vi "Vision.vi"() -> ()   [LabVIEW 2013]
uses:
  StateMachineStates 1.ctl
  <vilib>/DAQmx/read.llb/DAQmx Read (Counter DBL 1Chan 1Samp).vi
  <vilib>/Utility/file.llb/Write To Spreadsheet File (DBL).vi
  <vilib>/DAQmx/create/channels.llb/DAQmx Create Channel (CI-Pulse Width).vi
  <vilib>/DAQmx/miscellaneous.llb/DAQmx Fill In Error Info.vi
panel:
  in  "Stimulus delay (ms)":u32
  in  "N \n(calibration)":i32=5
  in  "Threshold\n (calibration)":dbl
  out "Pump calibration array":dbl[][](array[numeric])
  out "Calibrating":bool
  in  "Calibrate":bool
  out "current time":timestamp
  in  "Threshold":dbl=0.1 format="%#_13g"
  in  "Number of\ntrials to avg":i32=5
  in  "Pump mode":enum16{"Constant power", "Constant time"}(ring)
  in  "Target trigger\nrate (Hz)":dbl
  out "Pockels cell\nposition":dbl
  out "Waveplate\nposition":dbl
  out "Right\nposition":dbl
  out "Left\nposition":dbl
  in  "EEG timeout":i32
  out "Triggered":bool
  in  "Use EEG trigger?":bool
  in  "Entrainment":bool
  in  "Sound at \nstimulus end":bool
  in  "Manual \nvoltage (V)":dbl=2.6 format="%.2p"
  in  "Manual \nphoton #":i64=100
  out "L/R WP target":dbl
  out "List of axes":i32[](array[numeric])
  out "List of WP errors":bool[](array[boolean])
  out "WP error":bool
  out "appended array":dbl[][](array[numeric])
  out "Pump WP":dbl format="%.2f"
  in  "Target trial \nlength (ms)":dbl=500.0 format="%.2p"
  in  "Default pump \nWP angle":dbl=52.6
  in  "Pump WP":bool
  out "Photon time (ms)":dbl format="%.2f"
  in  "Interval (ms)":u32
  out "Repetition":dbl
  in  "Repetitions":dbl=1.0
  out "WP time (ms)":u32
  out "VISA Handle out":refnum<visa-resource-name>="ASRL5::INSTR"
  out "Initializing":bool
  out "Trial mode":enum16{"Single Photons", "LED", "Mixed LED"}(ring)
  in  "Frequency of LED trials\nfor Mixed mode":dbl=30.0
  out "Bright trial\nrequested":bool
  out "Observer Ready":bool
  in  "Bright/mixed mode \nLED voltage (V)":dbl=2.6 min=-3.0 max=4.0 format="%.2f"
  in  "GPIB address":string="15"
  in  "Period (ms)":i64=20
  in  "Pulse \nlength (ms)":dbl=50.0
  out "L/R WP":dbl format="%.2f"
  in  "Manually \ninitialize":bool
  in  "COM for WPs":u8=3
  out "Blocked trial #":i32
  out "Photon #":i32
  out "LED Voltage":dbl
  in  "Blocking requirements":cluster{"Value":dbl, " Number":i32}[](array[cluster])
  in  "Manual":bool
  in  "Path":path=path "C:/Users/lab/Dropbox/Research/Data/Vision"
  out "Counts 2":u32
  out "Counts 1":u32
  in  "Delay for APDs (ms)":u32
  in  "Counter 2":tag="Dev1/ctr1"
  in  "Counter 1":tag="Dev1/ctr0"
  out "Trial #":i32
  in  "Session Mode":enum16{"Single Photons", "LED", "Mixed"}(ring)=enum."Mixed"
  in  "Audio":bool=TRUE
  in  "Self-paced":bool
  out "Stimulus":bool
  out "Location Set":bool
  out "Stimulus \nlocation":string
  out "Waiting":bool
  out "Observer Responded":bool
  out "Response \ntime (ms)":dbl
  out "Observer \nchoice":string
  out "Confidence":i32
  in  "stop":bool
  in  "Next Trial":bool
  in  "Create New File":bool
  out "Subject #":string
  # "Instructions: Run VI. Enter blocking requirements, then press\nCreate New File. Initialize waveplates if necessary, and set\nhighlighted controls to desired values. Press Next Trial to begin."
  # "Researcher Interface"
  # "Settings for Blocking\nand Mixed Mode"
  # "(1)"
  # "Trial Options"
  # "Counter Options"
  # "Trial Information"
  # "EEG Options"
  # "Pump Settings"
  # "Waveplates"
  # "LED Options"
  # "(3)"
  # "(2)"
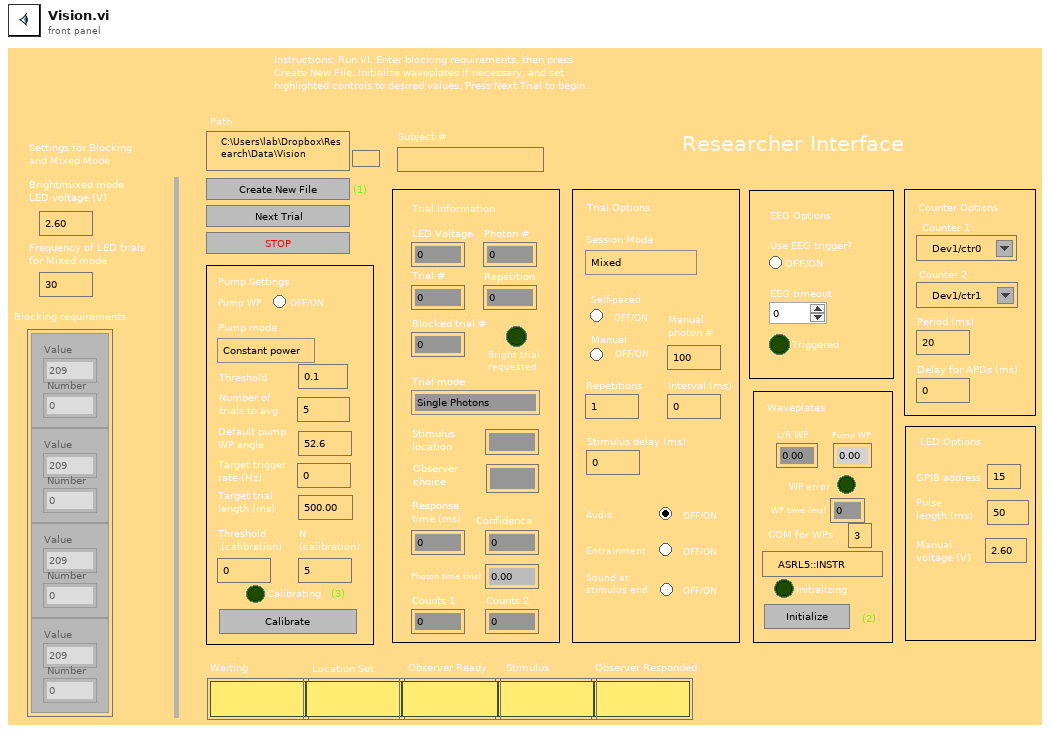
[diagram p1: front panel]
types:
  T1 = typedef "StateMachineStates 1.ctl" = enum16{"WaitResearcher", "Setup", "SetWP", "WaveplateError", "WaitObserverReady", "EEG", "Photons", "LED", "WaitObserverResponse", "CleanUp", "Stop"}
  T2 = enum16{"0", "1", "2", "3", "4", "5", "6", "7", "8", "9", "A", "B", "C", "D", "E", "F", "G", "H", "I", "J", "K", "L", "M", "N", "O", "P", "Q", "R", "S", "T", "U", "V", "W", "X", "Y", "Z", "F1", "F2", "F3", "F4", "F5", "F6", "F7", "F8", "F9", "F10", "F11", "F12", "F13", "F14", "F15", "ADD", "BACK", "BACKSLASH", "CAPITAL", "COMMA", "DECIMAL", "DELETE", "DIVIDE", "DOWN", "END", "EQUALS", "ESCAPE", "GRAVE (`)", "HOME", "INSERT", "LBRACKET", "LCONTROL", "LEFT", "L ALT", "LSHIFT", "LWIN", "MINUS", "MULTIPLY", "NEXT", "NUMLOCK", "NUMPAD_0", "NUMPAD_1", "NUMPAD_2", "NUMPAD_3", "NUMPAD_4", "NUMPAD_5", "NUMPAD_6", "NUMPAD_7", "NUMPAD_8", "NUMPAD_9", "PAUSE", "PERIOD", "PRIOR (PG UP)", "RBRACKET", "RCONTROL", "RETURN", "RIGHT", "R ALT", "RSHIFT", "RWIN", "SCROLL", "SEMICOLON", "SLASH", "SPACE", "SUBTRACT", "TAB", "UP", "ENTER (num pad)", "' (quote)"}
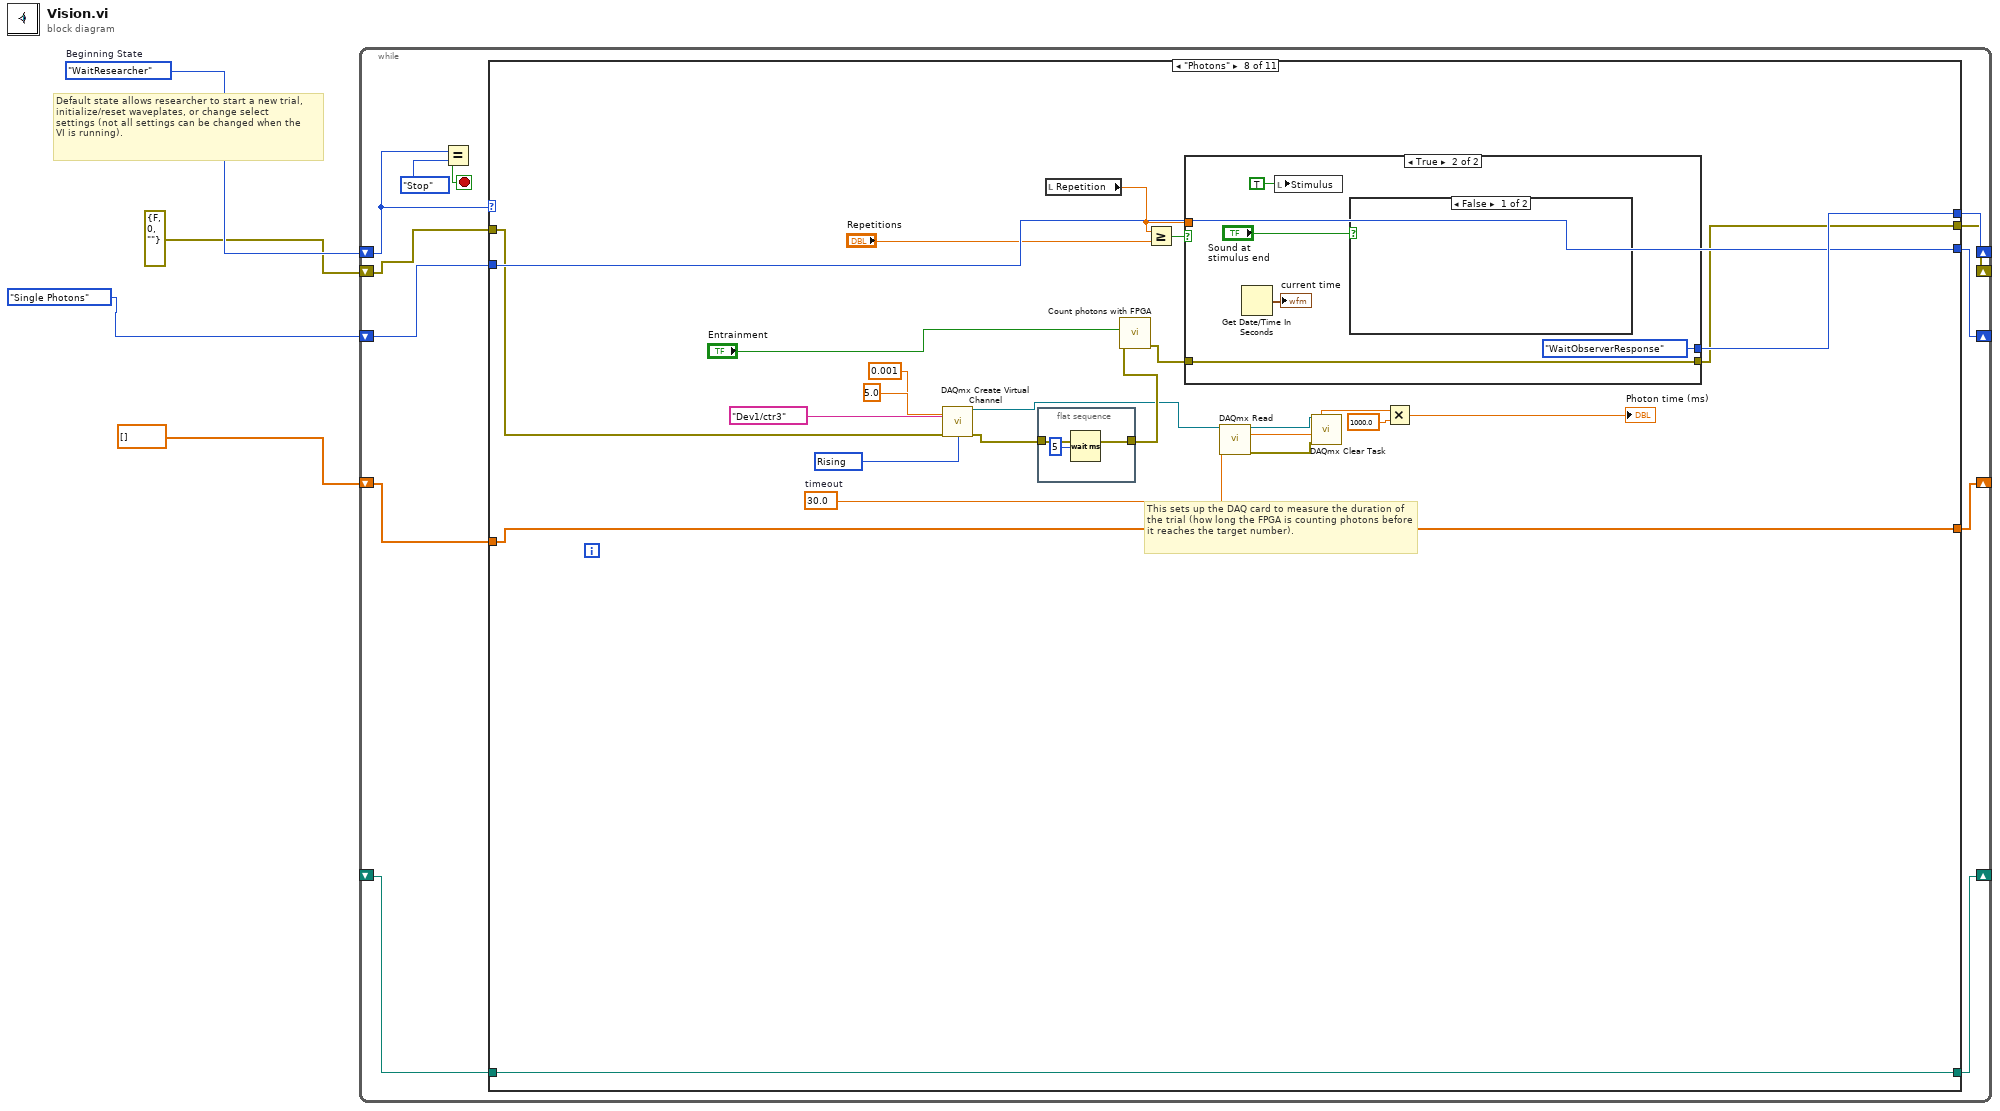
[diagram p0: block diagram]
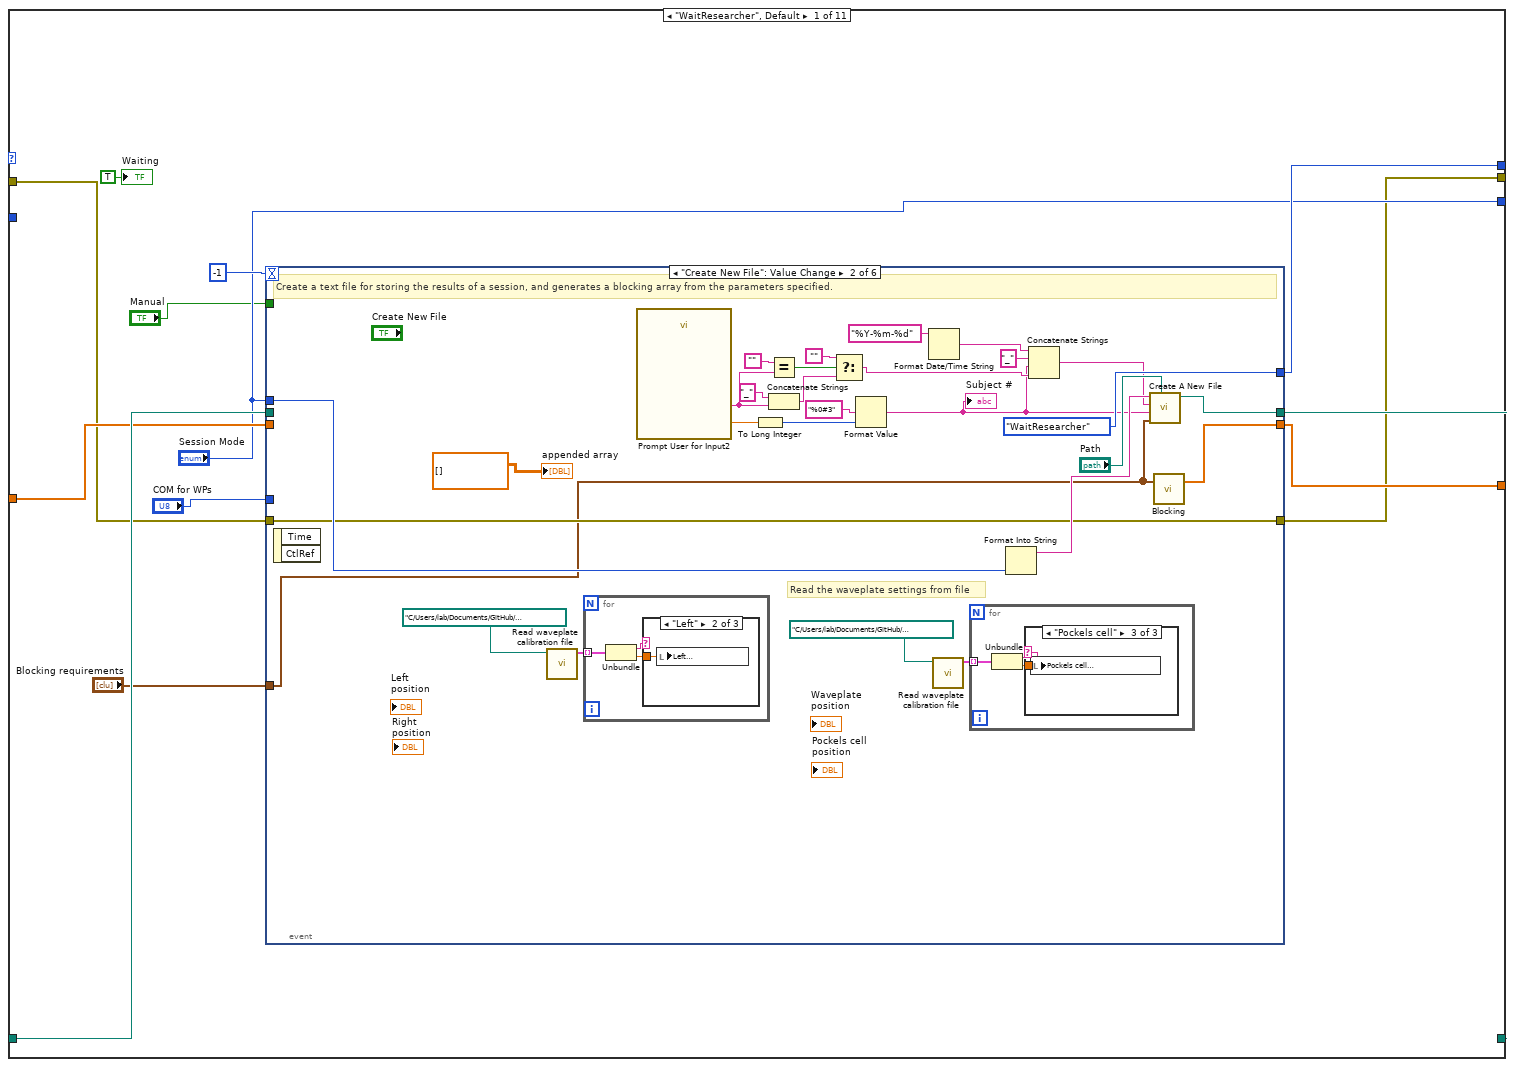
[diagram p2: hidden frame]
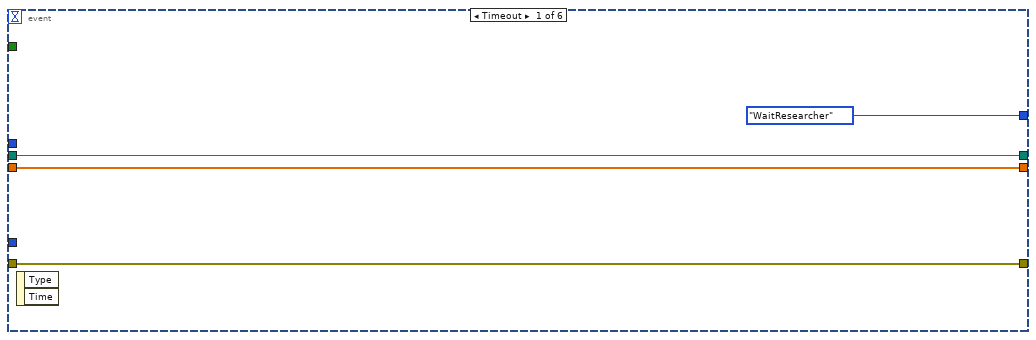
[diagram p3: hidden frame]
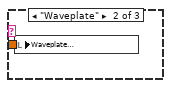
[diagram p5: hidden frame]
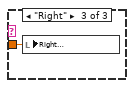
[diagram p7: hidden frame]
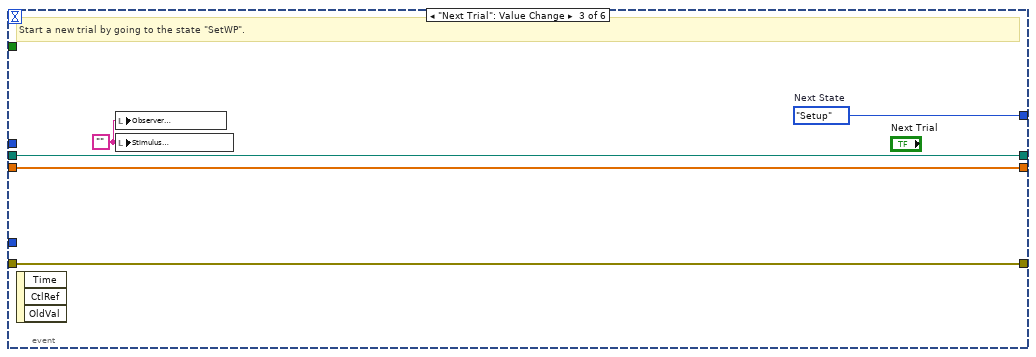
[diagram p8: hidden frame]
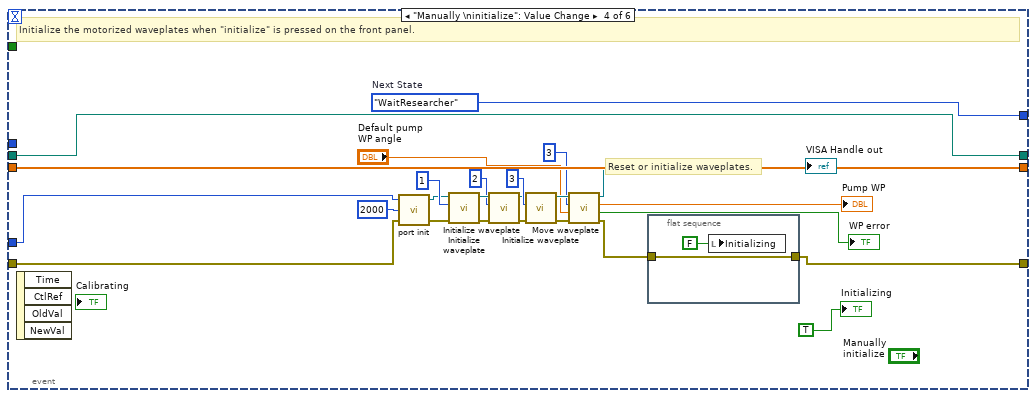
[diagram p9: hidden frame]
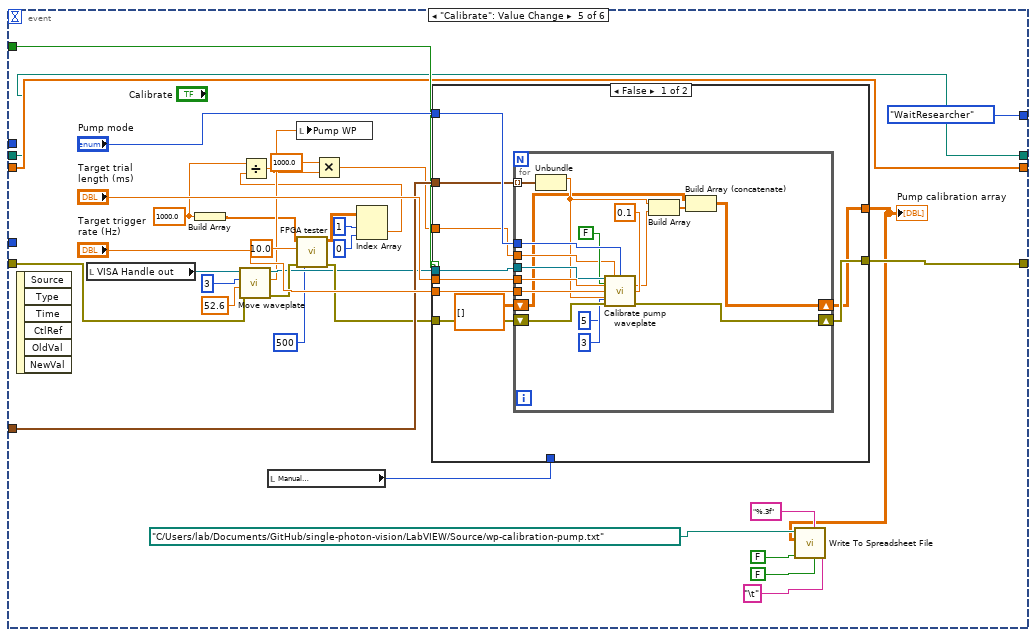
[diagram p10: hidden frame]
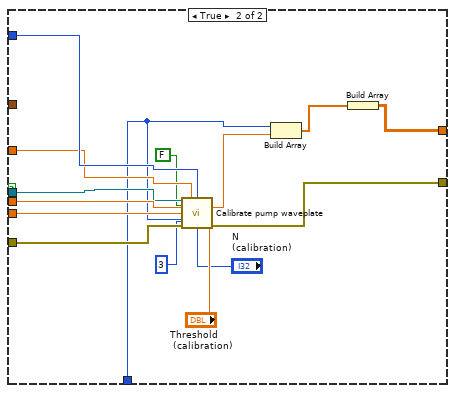
[diagram p11: hidden frame]
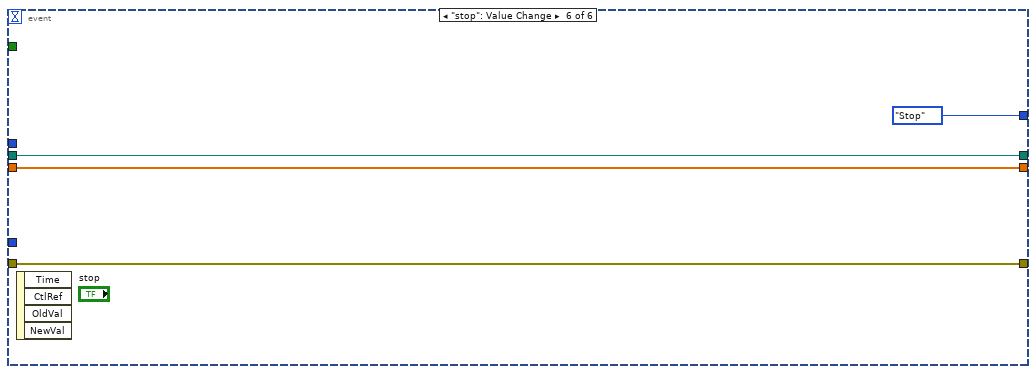
[diagram p12: hidden frame]
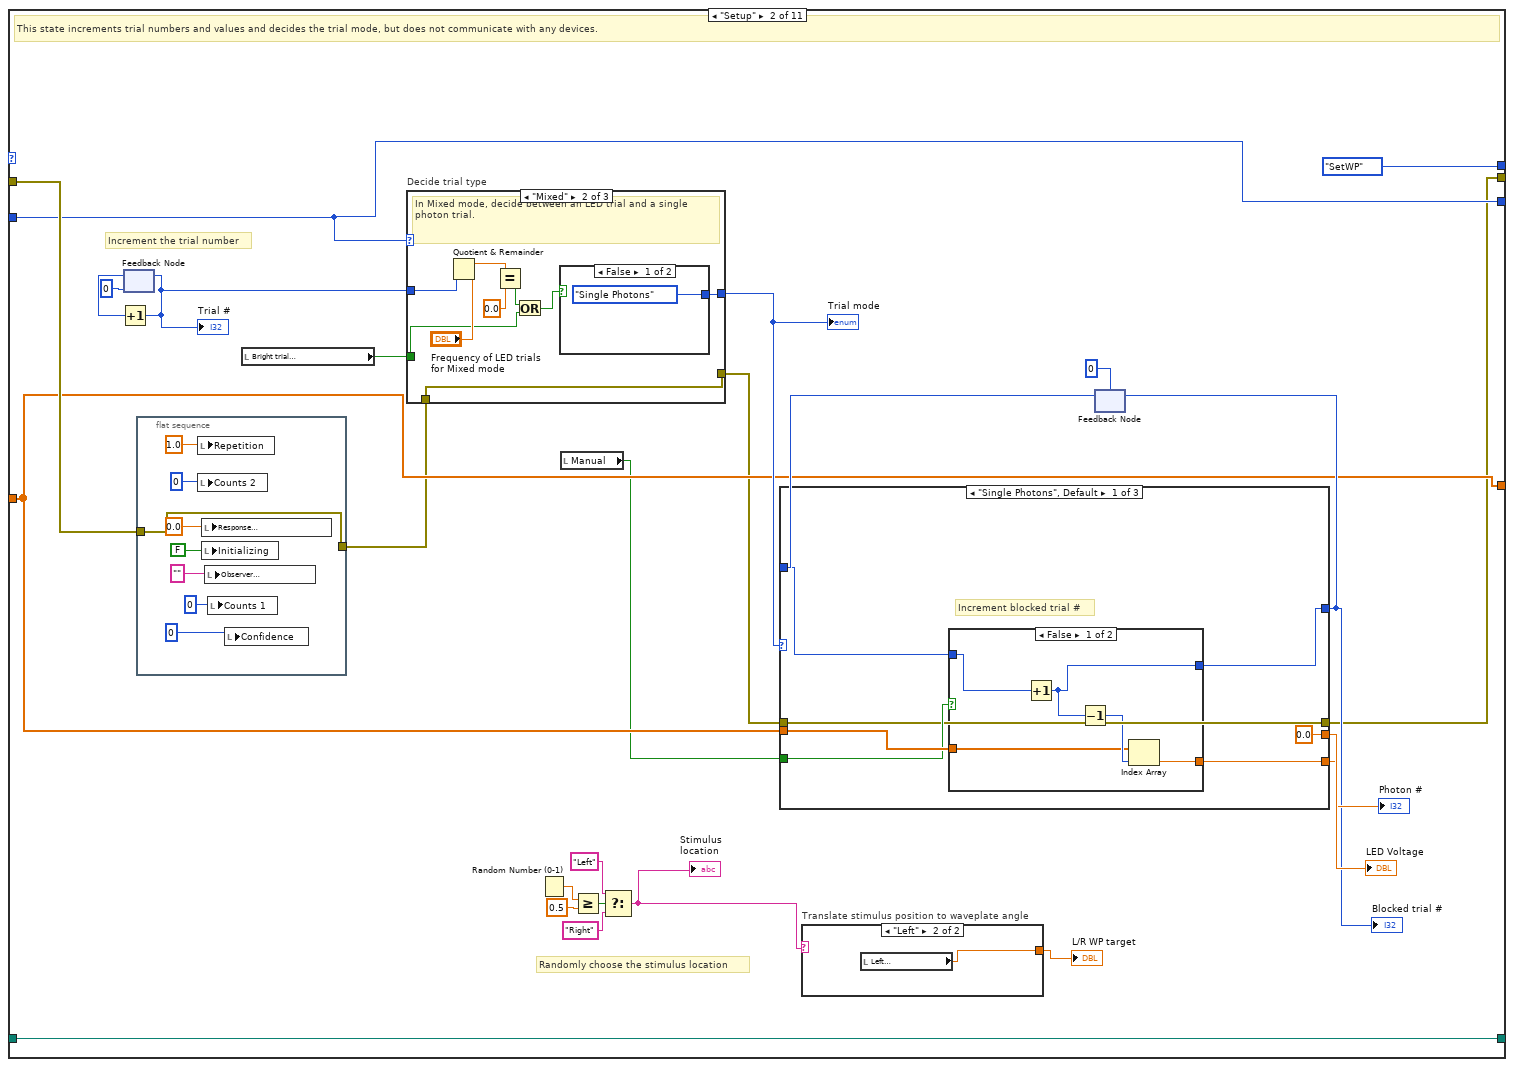
[diagram p13: hidden frame]
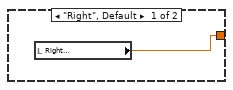
[diagram p14: hidden frame]
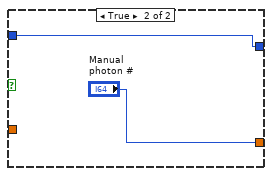
[diagram p15: hidden frame]
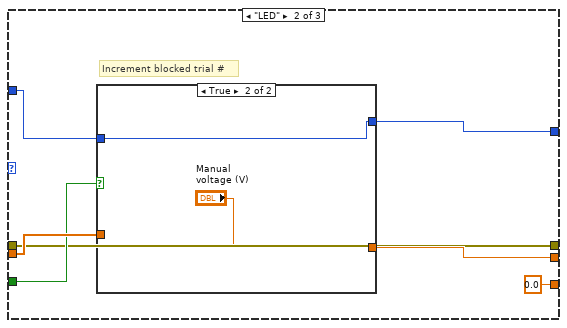
[diagram p16: hidden frame]
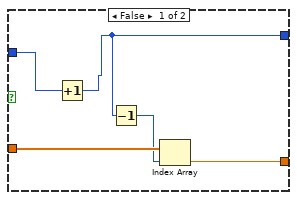
[diagram p17: hidden frame]
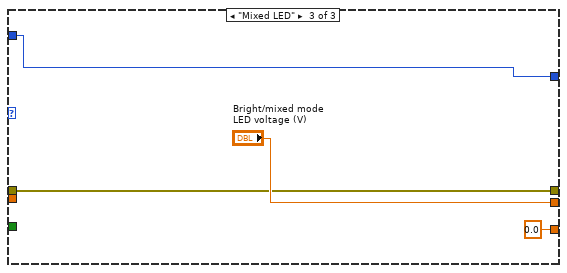
[diagram p18: hidden frame]
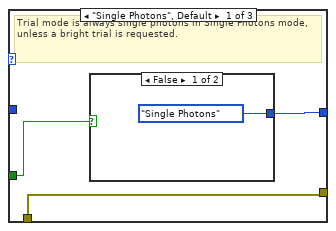
[diagram p19: hidden frame]
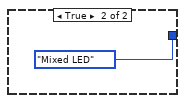
[diagram p20: hidden frame]
diagram:
  w4 = StateMachineStates_1."WaitResearcher"  # Beginning State
  # "Default state allows researcher to start a new trial,\ninitialize/reset waveplates, or change select\nsettings (not all settings can be changed when the\nVI is running)."
  n1 = while {
    shift-right: [w13] -> _
    shift-left: w4 -> [w14]
    shift-right: [w6] -> _
    shift-left: errorcluster {"status"=FALSE, "code"=0, "source"=""} ("error out") -> [w12]
    shift-right: [w11] -> _
    shift-left: enum16{"Single Photons", "LED", "Mixed"}."Single Photons" ("Mode") -> [w10]
    shift-right: [w9] -> _
    shift-left: _ -> [w5]
    shift-right: [w8] -> _
    shift-left: dbl[] [] ("Blocking array") -> [w7]
    stop <- w16 stop-if-true
    n2 = Equal?(x=w14, y=StateMachineStates_1."Stop" ("States")) -> (x = y?=w16:bool)
    n3 = case shown="\"Photons\"" w14 {
      selector: w14 -> [_ _ _ _ w497 _ _ _ _ _ _]
      tunnel: [w29 StateMachineStates_1."SetWP" ("Next State") w301 w443 w498 w539 StateMachineStates_1."WaitObserverResponse" ("Next State") w593 w610 w666 w705] -> w13
      tunnel: [w20 w193 w281 w440 w490 w541 w566 w589 w611 w657 w709] -> w6
      tunnel: w12 -> [w21 w210 w307 w444 w491 w541 w555 w575 w612 w656 w708]
      tunnel: ["Session Mode" w199 w319 w447 w495 w542 w562 w592 w617 w664 w712] -> w11
      tunnel: w10 -> [_ w199 w319 w447 w494 w542 w562 w592 w617 w664 w712]
      tunnel: [w26 w192 w320 w445 w493 w543 w559 w591 w616 w663 w711] -> w9
      tunnel: w5 -> [w25 w192 w320 w445 w493 w543 w559 w591 w616 w663 w711]
      tunnel: [w24 w198 w310 w446 w492 w544 w558 w590 w615 w661 w710] -> w8
      tunnel: w7 -> [w23 w198 w310 w446 w492 w544 w558 w590 w615 w661 w710]
      frame "WaitResearcher", Default {
        n4 = event shown="[1] \"Create New File\": Value Change" {
          selector: _ -> [_ _ _ _ _ _]
          dyn-events: _ -> [_ _ _ _ _ _]
          timeout: -1 -> [_ _ _ _ _ _]
          tunnel: [StateMachineStates_1."WaitResearcher" ("Next State") StateMachineStates_1."WaitResearcher" ("Next State") w72 w101 StateMachineStates_1."WaitResearcher" ("Next State") StateMachineStates_1."Stop" ("Next State")] -> w29
          tunnel: "Session Mode" -> [_ w57 _ _ _ _]
          tunnel: [w33 w52 w75 w100 w106 w183] -> w26
          tunnel: w25 -> [w33 _ w75 w100 w106 w183]
          tunnel: [w32 w55 w74 w98 w107 w182] -> w24
          tunnel: w23 -> [w32 _ w74 w98 w107 w182]
          tunnel: w21 -> [w31 w51 w73 w93 w128 w181]
          tunnel: [w31 w51 w73 w97 w134 w181] -> w20
          tunnel: "COM for WPs" -> [_ _ _ w94 _ _]
          tunnel: "Blocking requirements" -> [_ w34 _ _ w135 _]
          tunnel: "Manual" -> [_ _ _ _ w121 _]
          event Timeout {
            n5 = event-data() -> ()  [unwired: 1 in, 2 out]
          }
          event "Create New File": Value Change {
            # "Read the waveplate settings from file"
            # "Create a text file for storing the results of a session, and generates a blocking array from the parameters specified."
            n6 = event-data() -> ()  [unwired: 1 in, 2 out]
            n7 = call "Read waveplate calibration file.vi"("file path (dialog if empty)"=path "C:/Users/lab/Documents/GitHub/single-photon-vision/LabVIEW/Source/wp-calibration-lr.txt") -> ("Calibration array"=w37:cluster{"String":string, dbl}[])  [unwired: 9 in, 1 out]
            n8 = for {
              tunnel: w37 -> [w69] mode=indexing
              n9 = Unbundle(w69) -> ("String"=w68:string, w67:dbl)
              n10 = case shown="\"Left\"" w68 {
                tunnel: w67 -> [_ w70 w71]
                frame Default {
                }
                frame "Left" {
                  n11 = local write "Left\nposition"(w70) -> ()
                }
                frame "Right" {
                  n12 = local write "Right\nposition"(w71) -> ()
                }
              }
            }
            n13 = call "Prompt User for Input2"() -> ("Subject #"=w60:dbl, "Filename"=w46:string)  [unwired: 16 in, 2 out]
            n14 = To Long Integer(number=w60) -> (32bit integer=w42:i32)
            n15 = Equal?(x="", y=w46) -> (x = y?=w58:bool)
            n16 = Concatenate Strings("_" ("string"), w46) -> (w49:string)
            n17 = Select(t="", s=w58, f=w49) -> (s? t:f=w44:string)
            n18 = Format Value(format string="%0#3", value (0)=w42) -> (output string=w41:string)  [unwired: 1 in]
            "Subject #" <- w41
            n19 = Format Date/Time String(time format string (%c)="%Y-%m-%d") -> (date/time string=w47:string)  [unwired: 2 in]
            n20 = call "Read waveplate calibration file.vi"("file path (dialog if empty)"=path "C:/Users/lab/Documents/GitHub/single-photon-vision/LabVIEW/Source/wp-calibration-pc.txt") -> ("Calibration array"=w35:cluster{"String":string, dbl}[])  [unwired: 9 in, 1 out]
            n21 = for {
              tunnel: w35 -> [w64] mode=indexing
              n22 = Unbundle(w64) -> ("String"=w63:string, w62:dbl)
              n23 = case shown="\"Pockels cell\"" w63 {
                tunnel: w62 -> [_ w65 w66]
                frame Default {
                }
                frame "Waveplate" {
                  n24 = local write "Waveplate\nposition"(w65) -> ()
                }
                frame "Pockels cell" {
                  n25 = local write "Pockels cell\nposition"(w66) -> ()
                }
              }
            }
            n26 = Format Into String(w57) -> (resulting string=w56:string)  [unwired: 3 in, 1 out]
            n27 = Concatenate Strings(w47, "_" ("string"), w41, w44) -> (w53:string)
            n28 = call "Create A New File.vi"("Path in"="Path", "Blocking requirements"=w34, "Subject #"=w41, "Filename"=w53, "Mode"=w56) -> ("Path out"=w52:path)  [unwired: 6 in]
            n29 = call "Blocking.vi"("Blocking requirements"=w34) -> ("Blocking array"=w55:dbl[])  [unwired: 2 in]
            "appended array" <- dbl[][] []
          }
          event "Next Trial": Value Change {
            w72 = StateMachineStates_1."Setup"  # Next State
            w76 = ""
            # "Start a new trial by going to the state \"SetWP\"."
            n30 = event-data() -> ()  [unwired: 1 in, 3 out]
            n31 = local write "Observer \nchoice"(w76) -> ()
            n32 = local write "Stimulus \nlocation"(w76) -> ()
          }
          event "Manually \ninitialize": Value Change {
            w101 = StateMachineStates_1."WaitResearcher"  # Next State
            # "Reset or initialize waveplates."
            # "Initialize the motorized waveplates when \"initialize\" is pressed on the front panel."
            n33 = event-data() -> ()  [unwired: 1 in, 4 out]
            n34 = call "port init.vi"("error in"=w93, "Timeout (ms)"=u32 2000 ("Timeout (300 ms)"), "SerialPort"=w94) -> ("error out"=w92:errorcluster, "Visa Handle"=w91:refnum<visa-resource-name>)  [unwired: 1 in]
            n35 = call "Initialize waveplate.vi"("error in (no error)"=w92, "Axis in"=1, "VISA Handle in"=w91) -> ("error out"=w88:errorcluster, "VISA Refnum out"=w90:refnum<visa-resource-name>)  [unwired: 6 in, 1 out]
            n36 = call "Initialize waveplate.vi"("error in (no error)"=w88, "Axis in"=2, "VISA Handle in"=w90) -> ("error out"=w85:errorcluster, "VISA Refnum out"=w86:refnum<visa-resource-name>)  [unwired: 6 in, 1 out]
            n37 = call "Initialize waveplate.vi"("error in (no error)"=w85, "Axis in"=3, "VISA Handle in"=w86) -> ("error out"=w81:errorcluster, "VISA Refnum out"=w84:refnum<visa-resource-name>)  [unwired: 6 in, 1 out]
            n38 = call "Move waveplate.vi"("error in (no error)"=w81, "Angle"="Default pump \nWP angle", "Axis in"=3, "VISA Refnum in"=w84) -> ("error out"=w80:errorcluster, "WP Error"=→"WP error":bool, "Current position (units)"=→"Pump WP":dbl, "VISA Refnum out"=→"VISA Handle out":refnum<visa-resource-name>)  [unwired: 4 in]
            n39 = flat-sequence {
              tunnel: w80 -> [w103]
              tunnel: [w103] -> w97
              frame #0 {
                n40 = local write "Initializing"(FALSE ("Initializing waveplates")) -> ()
              }
            }
            "Initializing" <- TRUE ("Initializing waveplates")
          }
          event "Calibrate": Value Change {
            w113 = 1000.0 ("element")
            n41 = event-data() -> ()  [unwired: 1 in, 6 out]
            n42 = local read "VISA Handle out"() -> (w126:refnum<visa-resource-name>)
            n43 = Build Array(w113) -> (w114:dbl[])
            n44 = call "Move waveplate.vi"("error in (no error)"=w128, "Angle"=52.6, "Axis in"=3, "VISA Refnum in"=w126) -> ("error out"=w127:errorcluster, "Current position (units)"=w122:dbl, "VISA Refnum out"=w125:refnum<visa-resource-name>)  [unwired: 4 in, 1 out]
            n45 = local read "Manual \nphoton #"() -> (w120:i64)
            n46 = local write "Pump WP"(w122) -> ()
            n47 = call "FPGA tester.vi"("error in"=w127, "Delay"=u32 500, "Repetitions"=10.0, "Levels"=w114) -> ("error out"=w133:errorcluster, "Results"=w131:dbl[][])  [unwired: 2 in]
            n48 = Index Array(array=w131, index (row)=1, index (col)=0 ("disabled index (col)")) -> (element=w112:dbl)
            n49 = Divide(x=w113, y=w112) -> (x/y=w111:dbl)
            n50 = Multiply(x=1000.0, y=w111) -> (x*y=w109:dbl)
            n51 = case shown="False" w121 {
              tunnel: "Target trigger\nrate (Hz)" -> [w148 w180]
              tunnel: "Target trial \nlength (ms)" -> [w147 w179]
              tunnel: "Pump mode" -> [w146 w178]
              tunnel: w135 -> [w145 _]
              tunnel: [w144 w177] -> w134
              tunnel: w133 -> [w143 w176]
              tunnel: w109 -> [w142 w175]
              tunnel: w125 -> [w141 w174]
              tunnel: w120 -> [_ w173]
              tunnel: [w140 w168] -> w108
              frame False {
                n52 = for {
                  tunnel: w148 -> [w165]
                  tunnel: w147 -> [w164]
                  tunnel: w146 -> [w163]
                  tunnel: w145 -> [w162] mode=indexing
                  shift-right: [w160] -> w144
                  shift-left: w143 -> [w161]
                  tunnel: w141 -> [w159]
                  tunnel: w142 -> [w154]
                  shift-right: [w150] -> w140
                  shift-left: dbl[][] [] -> [w149]
                  n53 = Unbundle(w162) -> ("Value"=w153:dbl)  [unwired: 1 out]
                  n54 = call "Calibrate pump waveplate.vi"("VISA Refnum in"=w159, "Trigger rate \nat maximum"=w154, "Mode"=w163, "Trigger rate warnings?"=FALSE, "Target trial \nlength (ms)"=w164, "Target trigger rate"=w165, "Threshold"=0.1, "Photon #"=w153, "error in (no error)"=w161, "N"=5, "Axis in"=3) -> ("WP position"=w152:dbl, "error out"=w160:errorcluster)  [unwired: 1 in, 2 out]
                  n55 = Build Array(w153, w152) -> (w151:dbl[])
                  n56 = Build Array (concatenate)(w149, w151) -> (w150:dbl[][])
                }
              }
              frame True {
                n57 = call "Calibrate pump waveplate.vi"("VISA Refnum in"=w174, "Trigger rate \nat maximum"=w175, "Mode"=w178, "Trigger rate warnings?"=FALSE, "Target trial \nlength (ms)"=w179, "Target trigger rate"=w180, "Threshold"="Threshold\n (calibration)", "Photon #"=w173, "error in (no error)"=w176, "N"="N \n(calibration)", "Axis in"=3) -> ("WP position"=w170:dbl, "error out"=w177:errorcluster)  [unwired: 1 in, 2 out]
                n58 = Build Array(w173, w170) -> (w169:dbl[])
                n59 = Build Array(w169) -> (w168:dbl[][])
              }
            }
            "Pump calibration array" <- w108
            n60 = call-poly <vilib>:"Write To Spreadsheet File.vi"("delimiter (\\t)"="\t" ("delimiter (\\t)"), "transpose? (no:F)"=FALSE, "format (%.3f)"="%.3f", "append to file? (new file:F)"=FALSE, "2D data"=w108, "file path (dialog if empty)"=path "C:/Users/lab/Documents/GitHub/single-photon-vision/LabVIEW/Source/wp-calibration-pump.txt") -> ()  [unwired: 2 in, 1 out]
          }
          event "stop": Value Change {
            n61 = event-data() -> ()  [unwired: 1 in, 4 out]
          }
        }
        "Waiting" <- TRUE ("Waiting")
      }
      frame "Setup" {
        # "Randomly choose the stimulus location"
        # "Increment the trial number"
        # "This state increments trial numbers and values and decides the trial mode, but does not communicate with any devices."
        n62 = feedback #1(0 ("x+1")) -> (w209:i32)
        n63 = Increment(x=w209) -> (x+1=w207:i32)
        "Trial #" <- w207
        n64 = feedback-in #1(w207) -> ()
        n65 = flat-sequence {
          tunnel: w210 -> [w245]
          tunnel: [w245] -> w195
          frame #0 {
            n66 = local write "Repetition"(1.0 ("Repitition #")) -> ()
            n67 = local write "Counts 2"(u32 0 ("Counts 2")) -> ()
            n68 = local write "Response \ntime (ms)"(0.0 ("Response \ntime (ms)")) -> ()
            n69 = local write "Initializing"(FALSE ("Initializing waveplates")) -> ()
            n70 = local write "Observer \nchoice"("" ("Observer \nchoice")) -> ()
            n71 = local write "Counts 1"(u32 0 ("Counts 1")) -> ()
            n72 = local write "Confidence"(0 ("Confidence")) -> ()
          }
        }
        n73 = local read "Bright trial\nrequested"() -> (w200:bool)
        n74 = case "Decide trial type" shown="\"Mixed\"" w199 {
          tunnel: [w255 w265 w271] -> w206
          tunnel: w207 -> [_ w266 _]
          tunnel: w200 -> [w254 w259 w270]
          tunnel: w195 -> [w253 w258 w269]
          tunnel: [w253 w258 w269] -> w194
          frame "Single Photons", Default {
            # "Trial mode is always single photons in Single Photons mode, unless a bright trial is requested."
            n75 = case shown="False" w254 {
              tunnel: [enum16{"Single Photons", "LED", "Mixed LED"}."Single Photons" ("Mode") enum16{"Single Photons", "LED", "Mixed LED"}."Mixed LED" ("Mode")] -> w255
              frame False {
              }
              frame True {
              }
            }
          }
          frame "Mixed" {
            # "In Mixed mode, decide between an LED trial and a single photon trial."
            n76 = Quotient & Remainder(x=w266, y="Frequency of LED trials\nfor Mixed mode") -> (x-y*floor(x/y)=w263:dbl)  [unwired: 1 out]
            n77 = Equal?(x=w263, y=0.0) -> (x = y?=w261:bool)
            n78 = Or(x=w261, y=w259) -> (x .or. y?=w260:bool)
            n79 = case shown="False" w260 {
              tunnel: [enum16{"Single Photons", "LED", "Mixed LED"}."Single Photons" ("Mode") enum16{"Single Photons", "LED", "Mixed LED"}."Mixed LED" ("Mode")] -> w265
              frame False {
              }
              frame True {
              }
            }
          }
          frame "LED" {
            # "Trial mode is always LED in LED mode."
            n80 = case shown="False" w270 {
              tunnel: [enum16{"Single Photons", "LED", "Mixed LED"}."LED" ("Mode") enum16{"Single Photons", "LED", "Mixed LED"}."Mixed LED" ("Mode")] -> w271
              frame False {
              }
              frame True {
              }
            }
          }
        }
        "Trial mode" <- w206
        n81 = Random Number (0-1)() -> (number: 0 to 1=w191:dbl)
        n82 = local read "Manual"() -> (w197:bool)
        n83 = Greater Or Equal?(x=w191, y=0.5) -> (x >= y?=w189:bool)
        n84 = Select(t="Left", s=w189, f="Right") -> (s? t:f=w186:string)
        "Stimulus \nlocation" <- w186
        n85 = case "Translate stimulus position to waveplate angle" shown="\"Left\"" w186 {
          tunnel: [w211 w212] -> w185
          frame "Right", Default {
            n86 = local read "Right\nposition"() -> (w211:dbl)
          }
          frame "Left" {
            n87 = local read "Left\nposition"() -> (w212:dbl)
          }
        }
        "L/R WP target" <- w185
        n88 = feedback #2(0 ("x+1")) -> (w202:i32)
        n89 = case shown="\"Single Photons\", Default" w206 {
          tunnel: [w216 w232 w242] -> w201
          tunnel: w198 -> [w219 w233 _]
          tunnel: [0.0 ("Value") w231 "Bright/mixed mode \nLED voltage (V)"] -> w205
          tunnel: [w218 0.0 ("Value") 0.0 ("Value")] -> w204
          tunnel: w202 -> [w215 w229 w242]
          tunnel: w197 -> [w214 w228 _]
          tunnel: w194 -> [w213 w227 w241]
          tunnel: [w213 w227 w241] -> w193
          frame "Single Photons", Default {
            # "Increment blocked trial #"
            n90 = case shown="False" w214 {
              tunnel: w219 -> [w223 _]
              tunnel: [w222 "Manual \nphoton #"] -> w218
              tunnel: [w221 w225] -> w216
              tunnel: w215 -> [w220 w225]
              frame False {
                n91 = Increment(x=w220) -> (x+1=w221:i32)
                n92 = Decrement(x=w221) -> (x-1=w224:i32)
                n93 = Index Array(array=w223, index=w224) -> (element=w222:dbl)
              }
              frame True {
              }
            }
          }
          frame "LED" {
            # "Increment blocked trial #"
            n94 = case shown="True" w228 {
              tunnel: w233 -> [w238 _]
              tunnel: [w237 w239] -> w232
              tunnel: [w235 "Manual \nvoltage (V)"] -> w231
              tunnel: w229 -> [w234 w239]
              frame False {
                n95 = Increment(x=w234) -> (x+1=w237:i32)
                n96 = Decrement(x=w237) -> (x-1=w236:i32)
                n97 = Index Array(array=w238, index=w236) -> (element=w235:dbl)
              }
              frame True {
              }
            }
          }
          frame "Mixed LED" {
          }
        }
        "Photon #" <- w204
        "Blocked trial #" <- w201
        "LED Voltage" <- w205
        n98 = feedback-in #2(w201) -> ()
      }
      frame "SetWP" {
        # "Set waveplate/DG535/FPGA depending on trial mode."
        # "After moving waveplates, check for errors."
        # "Set the pump waveplate, if used"
        # "This state sets up the source for an upcoming trial, implementing waveplate settings, DG535 trigger settings, and FPGA settings."
        n99 = local read "L/R WP target"() -> (w285:dbl)
        n100 = local read "Photon #"() -> (w286:i32)
        n101 = local read "Target trial \nlength (ms)"() -> (w276:dbl)
        n102 = local read "Target trigger\nrate (Hz)"() -> (w277:dbl)
        n103 = local read "Pump calibration array"() -> (w274:dbl[][])
        n104 = local read "Trial mode"() -> (w283:enum16{"Single Photons", "LED", "Mixed LED"})
        n105 = flat-sequence {
          tunnel: w318 -> [w360]
          tunnel: w317 -> [w361]
          tunnel: [w361] -> w316
          tunnel: [w360] -> w315
          tunnel: [w359] -> w311
          tunnel: w285 -> [w358]
          tunnel: [w358] -> w284
          tunnel: w316 -> [w369]
          tunnel: w315 -> [w366]
          tunnel: [w363] -> w314
          tunnel: [w364] -> w313
          tunnel: [w371] -> w312
          tunnel: w311 -> [w371]
          tunnel: [w370] -> w296
          tunnel: [w365] -> w287
          tunnel: w284 -> [w368]
          tunnel: [w376] -> w279
          tunnel: [w377] -> w300
          tunnel: [w378] -> w321
          tunnel: w314 -> [w377]
          tunnel: w313 -> [w376]
          tunnel: w312 -> [w375]
          tunnel: w287 -> [w378]
          frame #0 {
            n106 = Tick Count (ms)() -> (millisecond timer value=w359:u32)
          }
          frame #1 {
            w367 = 1 ("Axis in")
            # "Ideally, this delay is set just slightly longer\nthan the time it takes the WP to move.\nThis ensures that the time needed for this\nstep is identical whether the WP setting\nis changed or not."
            n107 = Wait (ms)(milliseconds to wait=u32 3000) -> ()  [unwired: 1 out]
            n108 = call "Move waveplate.vi"("error in (no error)"=w369, "Angle"=w368, "Axis in"=w367, "VISA Refnum in"=w366) -> ("error out"=w363:errorcluster, "WP Error"=w362:bool, "Current position (units)"=w365:dbl, "VISA Refnum out"=w364:refnum<visa-resource-name>)  [unwired: 4 in]
            n109 = Bundle("WP Error"=w362, "Axis in"=w367) -> (w370:cluster{"WP Error":bool, "Axis in":i32})  [unwired: 1 in]
          }
          frame #2 {
            n110 = Tick Count (ms)() -> (millisecond timer value=w374:u32)
            n111 = Subtract(x=w374, y=w375) -> (x-y=→"WP time (ms)":u32)
          }
        }
        n112 = local read "appended array"() -> (w306:dbl[][])
        n113 = local read "VISA Handle out"() -> (w280:refnum<visa-resource-name>)
        n114 = Equal?(x=w283, y=enum16{"Single Photons", "LED", "Mixed LED"}."Single Photons") -> (x = y?=w303:bool)
        n115 = local read "Pump mode"() -> (w275:enum16{"Constant power", "Constant time"})
        n116 = And(x="Pump WP", y=w303) -> (x .and. y?=w302:bool)
        n117 = case shown="True" w302 {
          tunnel: w280 -> [w339 w344]
          tunnel: [w339 w347] -> w309
          tunnel: w307 -> [w338 w355]
          tunnel: [w338 w354] -> w308
          tunnel: w286 -> [_ w351]
          tunnel: w276 -> [_ w350]
          tunnel: w306 -> [_ w352]
          tunnel: [w336 w356] -> w297
          tunnel: w277 -> [_ w345]
          tunnel: w275 -> [_ w343]
          tunnel: w274 -> [_ w340]
          frame False {
            n118 = Bundle(FALSE, 3) -> (w336:cluster{bool, i32})  [unwired: 1 in]
          }
          frame True {
            n119 = call "Pump waveplate.vi"("VISA Refnum in"=w344, "Pump calibration array"=w340, "Mode"=w343, "Trigger rate warnings?"=FALSE, "Target trial \nlength (ms)"=w350, "Target trigger rate"=w345, "Threshold"="Threshold", "Photon #"=w351, "error in (no error)"=w355, "appended array"=w352, "N"="Number of\ntrials to avg", "Axis in"=3) -> ("VISA Refnum out"=w347:refnum<visa-resource-name>, "Current position (units)"=w348:dbl, "WP Error"=w346:bool, "error out"=w354:errorcluster)
            n120 = local write "Pump WP"(w348) -> ()
            n121 = Bundle("WP Error"=w346, 3) -> (w356:cluster{"WP Error":bool, i32})  [unwired: 1 in]
          }
        }
        n122 = local read "Waveplate\nposition"() -> (w278:dbl)
        n123 = case shown="\"LED\", Default" w283 {
          tunnel: w308 -> [w387 w399 w420]
          tunnel: [w380 w402 w424] -> w317
          tunnel: w309 -> [w390 w400 w422]
          tunnel: [w385 w395 w417] -> w318
          tunnel: [w391 w401 w423] -> w298
          tunnel: w278 -> [_ w393 w415]
          frame "Single Photons" {
            w389 = 2 ("Axis in")
            # "Convert number to a 16-bit\nunsigned integer."
            # "Transfer target count to FPGA as 4 sets of 4 bits."
            # "Set DG535 for triggering FPGA."
            # "Make sure WP is set for single photon trial."
            n124 = local read "Pockels cell\nposition"() -> (w379:dbl)
            n125 = call "Move waveplate.vi"("error in (no error)"=w387, "Angle"=w379, "Axis in"=w389, "VISA Refnum in"=w390) -> ("error out"=w386:errorcluster, "WP Error"=w388:bool, "VISA Refnum out"=w385:refnum<visa-resource-name>)  [unwired: 4 in, 1 out]
            n126 = Bundle("WP Error"=w388, "Axis in"=w389) -> (w391:cluster{"WP Error":bool, "Axis in":i32})  [unwired: 1 in]
            n127 = local read "Photon #"() -> (w383:i32)
            n128 = local read "GPIB address"() -> (w392:string)
            n129 = Number To Boolean Array(number=w383) -> (Boolean array=w382:bool[])
            n130 = call "Set DG535 for FPGA.vi"("error in (no error)"=w386, "GPIB address"=w392) -> ("error out"=w381:errorcluster)  [unwired: 9 in]
            n131 = call "Set FPGA target.vi"("error in (no error)"=w381, "Number of bits"=4, "Boolean array"=w382) -> ("error out"=w380:errorcluster)  [unwired: 8 in]
          }
          frame "LED", Default {
            w398 = 2 ("Axis in")
            # "Make sure WP is set for LED trial."
            # "Set relevent parameters on DG535 for LED flash."
            n132 = call "Move waveplate.vi"("error in (no error)"=w399, "Angle"=w393, "Axis in"=w398, "VISA Refnum in"=w400) -> ("error out"=w396:errorcluster, "WP Error"=w397:bool, "VISA Refnum out"=w395:refnum<visa-resource-name>)  [unwired: 4 in, 1 out]
            n133 = Bundle("WP Error"=w397, "Axis in"=w398) -> (w401:cluster{"WP Error":bool, "Axis in":i32})  [unwired: 1 in]
            n134 = local read "LED Voltage"() -> (w394:dbl)
            n135 = local read "GPIB address"() -> (w406:string)
            n136 = flat-sequence {
              tunnel: "Delay for APDs (ms)" -> [w412]
              tunnel: w406 -> [w411]
              tunnel: "Pulse \nlength (ms)" -> [w410]
              tunnel: w394 -> [w409]
              tunnel: w396 -> [w408]
              tunnel: [w407] -> w403
              tunnel: w403 -> [w413]
              tunnel: [w413] -> w402
              frame #0 {
                n137 = call "Set DG535 for LED.vi"("amplitude"=w409, "error in"=w408, "Delay (ms)"=w412, "Pulse length (ms)"=w410, "GPIB address"=w411) -> ("error out"=w407:errorcluster)  [unwired: 6 in]
              }
              frame #1 {
                n138 = Wait (ms)(milliseconds to wait=u32 100) -> ()  [unwired: 1 out]
              }
            }
          }
          frame "Mixed LED" {
            w421 = 2 ("Axis in")
            # "Set relevent parameters on DG535 for LED flash."
            # "Make sure WP is set for LED trial."
            n139 = local read "Bright/mixed mode \nLED voltage (V)"() -> (w416:dbl)
            n140 = call "Move waveplate.vi"("error in (no error)"=w420, "Angle"=w415, "Axis in"=w421, "VISA Refnum in"=w422) -> ("error out"=w419:errorcluster, "WP Error"=w418:bool, "VISA Refnum out"=w417:refnum<visa-resource-name>)  [unwired: 4 in, 1 out]
            n141 = Bundle("WP Error"=w418, "Axis in"=w421) -> (w423:cluster{"WP Error":bool, "Axis in":i32})  [unwired: 1 in]
            n142 = local read "Delay for APDs (ms)"() -> (w426:u32)
            n143 = local read "Pulse \nlength (ms)"() -> (w427:dbl)
            n144 = local read "GPIB address"() -> (w428:string)
            n145 = flat-sequence {
              tunnel: w426 -> [w433]
              tunnel: w428 -> [w432]
              tunnel: w427 -> [w431]
              tunnel: w416 -> [w430]
              tunnel: w419 -> [w429]
              tunnel: [w429] -> w425
              tunnel: w425 -> [w434]
              tunnel: [w434] -> w424
              frame #0 {
                n146 = call "Set DG535 for LED.vi"("amplitude"=w430, "Delay (ms)"=w433, "Pulse length (ms)"=w431, "GPIB address"=w432) -> ()  [unwired: 7 in, 1 out]
              }
              frame #1 {
                n147 = Wait (ms)(milliseconds to wait=u32 100) -> ()  [unwired: 1 out]
              }
            }
          }
        }
        n148 = Unbundle(w298) -> ("WP Error"=w294:bool, "Axis in"=w290:i32)
        n149 = Unbundle(w297) -> ("WP Error"=w293:bool, w289:i32)
        n150 = Unbundle(w296) -> ("WP Error"=w295:bool, "Axis in"=w291:i32)
        n151 = Compound Arithmetic op=OR(w295, w294, w293) -> (w299:bool)
        n152 = local write "WP error"(w299) -> ()
        n153 = Build Array(w295, w294, w293) -> (→"List of WP errors":bool[])
        n154 = local write "VISA Handle out"(w279) -> ()
        n155 = case shown="True" w299 {
          tunnel: [StateMachineStates_1."WaitObserverReady" ("Next State") StateMachineStates_1."WaveplateError" ("Next State")] -> w301
          tunnel: w300 -> [w324 w332]
          tunnel: [w324 w332] -> w282
          frame False {
            n156 = local write "Initializing"(FALSE ("WP Error")) -> ()
            "Location Set" <- TRUE ("Location Set")
          }
          frame True {
            n157 = call "Sound File to Sound Output.vi"("Volume"=100.0, "Number of Samples/Iteration"=10000, "Device ID"=u32 0, "File Path"=path "C:/Users/lab/Documents/GitHub/single-photon-vision/LabVIEW/Source/Windows Critical Stop.wav") -> ()
            n158 = local write "Initializing"(TRUE ("WP Error")) -> ()
          }
        }
        n159 = Build Array(w291, w290, w289) -> (→"List of axes":i32[])
        n160 = flat-sequence {
          tunnel: w282 -> [w323]
          tunnel: [w323] -> w281
          frame #0 {
            n161 = local write "Bright trial\nrequested"(FALSE ("Bright trial\nrequested")) -> ()
          }
        }
        "L/R WP" <- w321
      }
      frame "WaveplateError" {
        # "Resets waveplates in case of error in SetWP state."
        n162 = local read "VISA Handle out"() -> (w436:refnum<visa-resource-name>)
        n163 = call <vilib>:"Clear Errors.vi"("error in (no error)"=w444) -> ("error out"=w441:errorcluster)  [unwired: 6 in]
        n164 = local read "List of WP errors"() -> (w442:bool[])
        n165 = for {
          tunnel: w442 -> [w458] mode=indexing
          tunnel: w441 -> [w454]
          tunnel: [w453] -> w440
          tunnel: [w451] -> w438 mode=indexing
          shift-right: [w452] -> w439
          shift-left: w436 -> [w450]
          i -> [w456]
          n166 = local read "List of axes"() -> (w457:i32[])
          n167 = Index Array(array=w457, index=w456) -> (element=w455:i32)
          n168 = case shown="True" w458 {
            tunnel: w455 -> [_ w474]
            tunnel: w454 -> [w461 w475]
            tunnel: [w461 w471] -> w453
            tunnel: w450 -> [w460 w470]
            tunnel: [w460 w468] -> w452
            tunnel: [FALSE ("WP Error") w463] -> w451
            frame False {
            }
            frame True {
              n169 = local read "Pump WP"() -> (w465:bool)
              n170 = Not(x=w465) -> (.not. x?=w464:bool)
              n171 = call "Initialize waveplate.vi"("error in (no error)"=w475, "Axis in"=w474, "VISA Handle in"=w470) -> ("error out"=w472:errorcluster, "WP Error"=w462:bool, "VISA Refnum out"=w469:refnum<visa-resource-name>)  [unwired: 6 in]
              n172 = Equal?(x=3, y=w474) -> (x = y?=w467:bool)
              n173 = And(x=w464, y=w467) -> (x .and. y?=w466:bool)
              n174 = case shown="True" w466 {
                tunnel: w472 -> [w478 w483]
                tunnel: [w478 w482] -> w471
                tunnel: w469 -> [w477 w481]
                tunnel: [w477 w480] -> w468
                tunnel: [w476 w479] -> w463
                tunnel: w462 -> [w476 _]
                frame False {
                }
                frame True {
                  n175 = local read "Default pump \nWP angle"() -> (w485:dbl)
                  n176 = call "Move waveplate.vi"("error in (no error)"=w483, "Angle"=w485, "Axis in"=3, "VISA Refnum in"=w481) -> ("error out"=w482:errorcluster, "WP Error"=w479:bool, "Current position (units)"=w486:dbl, "VISA Refnum out"=w480:refnum<visa-resource-name>)  [unwired: 4 in]
                  n177 = local write "Pump WP"(w486) -> ()
                }
              }
            }
          }
        }
        n178 = local write "VISA Handle out"(w439) -> ()
        n179 = Or Array Elements(Boolean array=w438) -> (logical OR=w437:bool)
        n180 = case shown="True" w437 {
          tunnel: [StateMachineStates_1."SetWP" ("Next State") StateMachineStates_1."WaveplateError" ("Next State")] -> w443
          frame False {
          }
          frame True {
          }
        }
      }
      frame "WaitObserverReady" {
        # "Wait for the observer to trigger the beginning of a trial by pressing the spacebar, then go to a stimulus-producing state determined by \"session mode\" on the front panel."
        n181 = flat-sequence {
          tunnel: [w500] -> w496
          tunnel: w491 -> [w500]
          tunnel: w497 -> [w511]
          tunnel: w496 -> [w509]
          tunnel: w494 -> [w504]
          tunnel: [w505] -> w489
          tunnel: [w512] -> w488
          tunnel: [w508] -> w487
          tunnel: [w535] -> w495
          tunnel: [w536] -> w498
          tunnel: [w537] -> w490
          tunnel: w489 -> [w537]
          tunnel: w488 -> [w536]
          tunnel: w487 -> [w535]
          frame #0 {
            n182 = local read "Bright/mixed mode \nLED voltage (V)"() -> (w499:dbl)
            n183 = local read "LED Voltage"() -> (w501:dbl)
            n184 = call "Play sound start trial.vi"("LED Voltage"=w501, "Bright/mixed mode \nLED voltage (V)"=w499) -> ()  [unwired: 10 in]
          }
          frame #1 {
            n185 = local read "Trial mode"() -> (w503:enum16{"Single Photons", "LED", "Mixed LED"})
            n186 = call "Query Keyboard.vi"("error in (no error)"=w509, "Stop?"=FALSE) -> ("error out"=w506:errorcluster, "element"=w510:T2)  [unwired: 8 in]
            n187 = case shown="\"SPACE\"" w510 {
              tunnel: [StateMachineStates_1."WaitObserverReady" ("Next State") w522 StateMachineStates_1."WaitObserverReady" ("Next State")] -> w512
              tunnel: w511 -> [_ _ _]
              tunnel: [w515 w521 w532] -> w508
              tunnel: w504 -> [w515 w521 w532]
              tunnel: w506 -> [w514 w520 w529]
              tunnel: [w514 w520 w529] -> w505
              tunnel: w503 -> [_ w519 _]
              tunnel: [FALSE ("Observer Ready") TRUE ("Observer Ready") FALSE ("Observer Ready")] -> w502
              frame "1", Default {
              }
              frame "SPACE" {
                # "If the subject presses SPACE, move to the appropriate stimulus-producing mode (either Photons, Detectors, or LED)."
                n188 = case shown="False" "Use EEG trigger?" {
                  tunnel: [w524 w528] -> w522
                  tunnel: w519 -> [w523 _]
                  frame False {
                    n189 = case shown="\"Single Photons\", Default" w523 {
                      tunnel: [w525 w526 w527] -> w524
                      frame "Single Photons", Default {
                        w525 = StateMachineStates_1."Photons"  # Next State
                      }
                      frame "LED" {
                        w526 = StateMachineStates_1."LED"  # Next State
                      }
                      frame "Mixed LED" {
                        w527 = StateMachineStates_1."LED"  # Next State
                      }
                    }
                  }
                  frame True {
                    w528 = StateMachineStates_1."Photons"  # Next State
                  }
                }
              }
              frame "NUMPAD_0" {
                # "If the subject presses 0, set the \"bright trial requested\" flag and keep waiting for a response"
                "Bright trial\nrequested" <- TRUE ("Bright trial\nrequested")
              }
            }
            "Observer Ready" <- w502
          }
          frame #2 {
            n190 = Wait (ms)(milliseconds to wait="Stimulus delay (ms)") -> ()  [unwired: 1 out]
          }
        }
      }
      frame "EEG" {
        # "Wait for an EEG trigger, then go to the appropriate stimulus-producing state."
        n191 = call "EEGstatus.vi"() -> ("Is minima found?"=w540:bool)  [unwired: 11 in]
        n192 = local write "Triggered"(w540) -> ()
        n193 = event shown="[0] Timeout" {
          selector: _ -> [_ _]
          dyn-events: _ -> [_ _]
          timeout: "EEG timeout" -> [_ _]
          tunnel: [w549 w551] -> w539
          event Timeout {
            w549 = StateMachineStates_1."WaitObserverReady"  # Next State
            n194 = event-data() -> ()  [unwired: 1 in, 3 out]
            n195 = call "Sound File to Sound Output.vi"("Volume"=100.0, "Number of Samples/Iteration"=10000, "Device ID"=u32 0, "File Path"=path "C:/Users/lab/Dropbox/Vision software/Source/Windows Critical Stop.wav") -> ()
          }
          event "Triggered": Value Change {
            n196 = event-data() -> ()  [unwired: 1 in, 6 out]
            n197 = local read "Trial mode"() -> (w550:enum16{"Single Photons", "LED", "Mixed LED"})
            n198 = case shown="\"Single Photons\", Default" w550 {
              tunnel: [w552 w553 w554] -> w551
              frame "Single Photons", Default {
                w552 = StateMachineStates_1."Photons"  # Next State
              }
              frame "LED" {
                w553 = StateMachineStates_1."LED"  # Next State
              }
              frame "Mixed LED" {
                w554 = StateMachineStates_1."LED"  # Next State
              }
            }
          }
        }
      }
      frame "LED" {
        # "Flash LED while reading out counts from two single-photon detectors."
        n199 = call "flashLED_DG535andcount.vi"("error in"=w555, "GPIB address"="GPIB address", "Period"="Period (ms)", "Counter 2"="Counter 2", "Counter 1"="Counter 1") -> ("Counts 2"=→"Counts 2":u32, "Counts 1"=→"Counts 1":u32, "error out"=w565:errorcluster)  [unwired: 4 in]
        n200 = flat-sequence {
          tunnel: w565 -> [w568]
          tunnel: [w568] -> w566
          frame #0 {
            "Stimulus" <- TRUE ("Stimulus")
          }
        }
      }
      frame "Photons" {
        w582 = 30.0  # timeout
        w573 = 10280 items=["Rising"=10280, "Falling"=10171] ("Starting Edge")
        # "This sets up the DAQ card to measure the duration of the trial (how long the FPGA is counting photons before it reaches the target number)."
        n201 = call-poly <vilib>:"DAQmx Create Virtual Channel.vi"("maximum value"=5.0 ("Maximum Value (sec)"), "minimum value"=0.001 ("Minimum Value (sec)"), "counter"=tag "Dev1/ctr3" ("Physical Channel"), "error in"=w575, "starting edge"=w573) -> ("task out"=w570:refnum<k21>, "error out"=w572:errorcluster)  [unwired: 9 in]
        n202 = flat-sequence {
          tunnel: w572 -> [w595]
          tunnel: [w595] -> w571
          frame #0 {
            n203 = Wait (ms)(milliseconds to wait=u32 5) -> ()  [unwired: 1 out]
          }
        }
        n204 = local read "Repetition"() -> (w586:dbl)
        n205 = call "Count photons with FPGA.vi"("error in (no error)"=w571, "Entrainment"="Entrainment") -> ("error out"=w585:errorcluster)  [unwired: 9 in]
        n206 = Greater Or Equal?(x=w586, y="Repetitions") -> (x >= y?=w588:bool)
        n207 = case shown="True" w588 {
          tunnel: [StateMachineStates_1."Photons" ("States") StateMachineStates_1."WaitObserverResponse" ("States")] -> w593
          tunnel: w585 -> [w599 w604]
          tunnel: [w599 w604] -> w589
          tunnel: w586 -> [w598 _]
          frame False {
            n208 = Increment(x=w598) -> (x+1=→"Repetition":dbl)
            n209 = Wait (ms)(milliseconds to wait="Interval (ms)") -> ()  [unwired: 1 out]
          }
          frame True {
            n210 = Get Date/Time In Seconds() -> (seconds since 1Jan1904=→"current time":timestamp)
            n211 = local write "Stimulus"(TRUE ("Counts Taken")) -> ()
            n212 = case shown="False" "Sound at \nstimulus end" {
              frame False {
              }
              frame True {
                n213 = call "Sound File to Sound Output.vi"("Volume"=100.0, "Number of Samples/Iteration"=10000, "Device ID"=u32 0, "File Path"=path "C:/Users/lab/Documents/GitHub/single-photon-vision/LabVIEW/Source/Speech Misrecognition.wav") -> ()
              }
            }
          }
        }
        n214 = call-poly <vilib>:"DAQmx Read.vi"("task/channels in"=w570, "timeout"=w582) -> ("task out"=w580:refnum<k21>, "data"=w584:dbl, "error out"=w581:errorcluster)  [unwired: 11 in]
        n215 = call <vilib>:"DAQmx Clear Task.vi"("task in"=w580, "error in"=w581) -> ()  [unwired: 13 in, 1 out]
        n216 = Multiply(x=w584, y=1000.0) -> (x*y=→"Photon time (ms)":dbl)
      }
      frame "WaitObserverResponse" {
        n217 = flat-sequence {
          tunnel: w612 -> [w618]
          tunnel: [w618] -> w613
          tunnel: [w619] -> w614
          tunnel: w613 -> [w619]
          tunnel: [w650] -> w610
          tunnel: [w644] -> w611
          tunnel: w614 -> [w644]
          frame #0 {
          }
          frame #1 {
            n218 = while {
              stop <- w623 stop-if-true
              n219 = call "Query Keyboard.vi"("Stop?"=FALSE) -> ("element"=w621:T2)  [unwired: 9 in, 1 out]
              n220 = case shown="\"D\", \"F\", \"S\"" w621 {
                tunnel: ["Left" w632 "Right"] -> w622
                frame "D", "F", "S" {
                }
                frame Default {
                  n221 = local read "Observer \nchoice"() -> (w632:string)
                }
                frame "J".."L" {
                }
              }
              "Observer \nchoice" <- w622
              n222 = case shown="\"S\"" w621 {
                tunnel: [0 1 2 3 3 2 1] -> w627
                frame Default {
                }
                frame "S" {
                }
                frame "D" {
                }
                frame "F" {
                }
                frame "J" {
                }
                frame "K" {
                }
                frame "L" {
                }
              }
              n223 = case shown="\"0\", Default" w621 {
                tunnel: [FALSE TRUE] -> w625
                frame "0", Default {
                }
                frame "SPACE" {
                }
              }
              n224 = local read "Confidence"() -> (w626:i32)
              n225 = Equal To 0?(x=w627) -> (x = 0?=w629:bool)
              n226 = Greater Than 0?(x=w626) -> (x > 0?=w624:bool)
              n227 = And(x=w629, y=w624) -> (x .and. y?=w628:bool)
              n228 = And(x=w625, y=w624) -> (x .and. y?=w623:bool)
              n229 = Select(t=w626, s=w628, f=w627) -> (s? t:f=w630:i32)
              n230 = local write "Confidence"(w630) -> ()
            }
          }
          frame #2 {
            w650 = StateMachineStates_1."CleanUp"  # Next State
            n231 = local read "current time"() -> (w643:timestamp)
            n232 = Get Date/Time In Seconds() -> (seconds since 1Jan1904=w648:timestamp)
            n233 = Subtract(x=w648, y=w643) -> (x-y=w647:dbl)
            n234 = Multiply(x=w647, y=1000.0) -> (x*y=→"Response \ntime (ms)":dbl)
            "Observer Responded" <- TRUE ("Boolean 3")
          }
        }
      }
      frame "CleanUp" {
        # "Reset indicators"
        # "Write data from trial to file."
        n235 = local read "Manual"() -> (w652:bool)
        n236 = local read "Stimulus \nlocation"() -> (w654:string)
        n237 = local read "Observer \nchoice"() -> (w651:string)
        n238 = local read "Blocked trial #"() -> (w653:i32)
        n239 = flat-sequence {
          tunnel: w654 -> [w683]
          tunnel: w651 -> [w682]
          tunnel: w663 -> [w681]
          tunnel: w656 -> [w679]
          tunnel: [w679] -> w655
          frame #0 {
            n240 = local read "Subject #"() -> (w668:string)
            n241 = Equal?(x=w683, y=w682) -> (x = y?=w685:bool)
            n242 = local read "Trial #"() -> (w672:i32)
            n243 = local read "Counts 2"() -> (w670:u32)
            n244 = local read "Counts 1"() -> (w669:u32)
            n245 = local read "Confidence"() -> (w671:i32)
            n246 = local read "Photon #"() -> (w678:i32)
            n247 = local read "Response \ntime (ms)"() -> (w684:dbl)
            n248 = local read "Photon time (ms)"() -> (w677:dbl)
            n249 = local read "LED Voltage"() -> (w680:dbl)
            n250 = local read "Pump WP"() -> (w673:dbl)
            n251 = call "Prepare data and write to file.vi"("Photon time (ms)"=w677, "String"=w683, "Confidence"=w671, "Photon #"=w678, "Pump WP"=w673, "Observer choice"=w682, "LED Voltage"=w680, "Response \ntime (ms)"=w684, "Path in"=w681, "Boolean"=w685, 10:w672, "Counts in"=w669, "Subject #"=w668, "Counts 1"=w670) -> ()  [unwired: 6 in]
            n252 = feedback #3(dbl[][] []) -> (w676:dbl[][])
            n253 = Build Array(w678, w677, w673) -> (w675:dbl[])
            n254 = Build Array (concatenate)(w675, w676) -> (w674:dbl[][])
            n255 = local write "appended array"(w674) -> ()
            n256 = feedback-in #3(w674) -> ()
          }
        }
        n257 = Array Size(array=w661) -> (size(s)=w660:i32)
        n258 = call "Play sound right wrong.vi"("Audio"="Audio", "String"=w654, "Observer choice"=w651) -> ()  [unwired: 9 in]
        n259 = Equal?(x=w660, y=w653) -> (x = y?=w659:bool)
        n260 = Not(x=w652) -> (.not. x?=w662:bool)
        n261 = And(x=w662, y=w659) -> (x .and. y?=w658:bool)
        n262 = case shown="False" w658 {
          tunnel: [w690 w699] -> w666
          tunnel: w652 -> [_ _]
          frame False {
            # "Display a message and\nswitch to manual mode\nif end of blocked trials\nis reached."
            n263 = case shown="True" "Self-paced" {
              tunnel: [w692 w696] -> w690
              frame False {
                n264 = call "Display Message to User"() -> ("OK"=w691:bool)  [unwired: 10 in, 1 out]
                n265 = case shown="True" w691 {
                  tunnel: [w693 w695] -> w692
                  frame False {
                    w693 = StateMachineStates_1."CleanUp"  # Next State
                  }
                  frame True {
                    w695 = StateMachineStates_1."WaitResearcher"  # Next State
                    n266 = local write "Observer Responded"(FALSE ("Observer Responded")) -> ()
                  }
                }
              }
              frame True {
                w696 = StateMachineStates_1."Setup"  # Next State
                # "Skip \"WaitingResearcher\" mode if trials are self-paced."
                n267 = local write "Observer Responded"(FALSE ("Observer Responded")) -> ()
              }
            }
          }
          frame True {
            n268 = local write "Self-paced"(FALSE ("Self-paced")) -> ()
            n269 = call "Display Message to User2"() -> ("OK"=w700:bool)  [unwired: 10 in, 1 out]
            n270 = case shown="False" w700 {
              tunnel: [w702 w704] -> w699
              frame False {
                w702 = StateMachineStates_1."CleanUp"  # Next State
              }
              frame True {
                w704 = StateMachineStates_1."WaitResearcher"  # Next State
                n271 = local write "Observer Responded"(FALSE ("Observer Responded")) -> ()
              }
            }
            n272 = local write "Manual"(TRUE ("Manual")) -> ()
          }
        }
        n273 = flat-sequence {
          tunnel: [w686] -> w657
          tunnel: w655 -> [w686]
          frame #0 {
            w688 = FALSE ("LC")
            n274 = local write "LED Voltage"(0.0 ("LED Voltage")) -> ()
            n275 = local write "Location Set"(w688) -> ()
            n276 = local write "Waiting"(w688) -> ()
            n277 = local write "Stimulus"(w688) -> ()
            n278 = local write "Observer Ready"(w688) -> ()
          }
        }
      }
      frame "Stop" {
        n279 = flat-sequence {
          tunnel: w708 -> [w714]
          tunnel: [w715] -> w707
          tunnel: w707 -> [w717]
          tunnel: [w717] -> w706
          tunnel: [w719] -> w709
          tunnel: w706 -> [w719]
          tunnel: [StateMachineStates_1."Stop" ("Next State")] -> w705
          frame #0 {
            # "Close waveplate session."
            n280 = local read "VISA Handle out"() -> (w713:refnum<visa-resource-name>)
            n281 = call "smc100_close.vi"("error in"=w714, "VISA Handle in"=w713) -> ("error out"=w715:errorcluster)  [unwired: 3 in]
          }
          frame #1 {
            w716 = FALSE ("LC")
            # "Reset indicator lights."
            n282 = local write "Stimulus"(w716) -> ()
            n283 = local write "Location Set"(w716) -> ()
            n284 = local write "Observer Responded"(w716) -> ()
            n285 = local write "Waiting"(w716) -> ()
            n286 = local write "Observer Ready"(w716) -> ()
          }
          frame #2 {
          }
        }
      }
    }
  }
